vi "F Dwf Digital Can Rx.vi"(0 "hdwf":i32, 1 "pvID":i32, 2 "pfExtended":i32, 3 "pfRemote":i32, 4 "pcDLC":i32, 5 "rgRX":string, 6 "cRX":i32, 7 "error in (no error)":errorcluster, 8 "pvStatus":i32) -> (18 "pvStatus out":i32, 20 "function return":i32, 21 "pvID out":i32, 22 "pfExtended out":i32, 23 "pfRemote out":i32, 24 "pcDLC out":i32, 25 "rgRX out":string, 27 "error out":errorcluster)   [LabVIEW 2021, in "Olasdwf.lvlib"]
doc: "DWFAPI int FDwfDigitalCanRx(HDWF hdwf, int *pvID, int *pfExtended, int *pfRemote, int *pcDLC, unsigned char *rgRX, int cRX, int *pvStatus);"
uses:
  Olasdwf.lvlib
  Windows/System32/dwf.dll
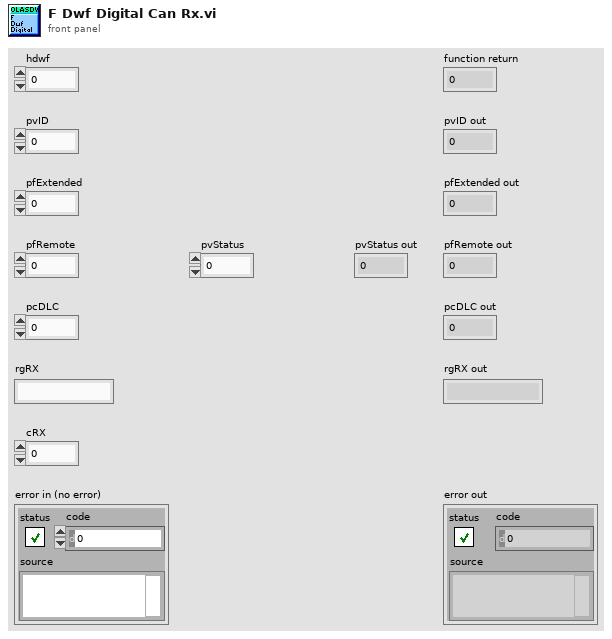
[diagram p1: front panel]
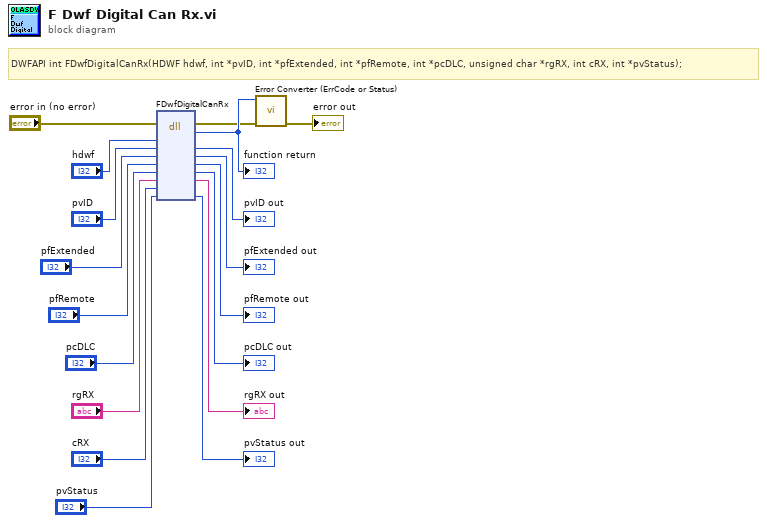
[diagram p0: block diagram]
diagram:
  # "DWFAPI int FDwfDigitalCanRx(HDWF hdwf, int *pvID, int *pfExtended, int *pfRemote, int *pcDLC, unsigned char *rgRX, int cRX, int *pvStatus);"
  n1 = dll-call lib="/Windows/System32/dwf.*" fn="FDwfDigitalCanRx"(error in="error in (no error)", "hdwf"="hdwf", "pvID"="pvID", "pfExtended"="pfExtended", "pfRemote"="pfRemote", "pcDLC"="pcDLC", "rgRX"="rgRX", "cRX"="cRX", "pvStatus"="pvStatus") -> (error out=w2:errorcluster, w18:i32, "pvID"=→"pvID out":i32, "pfExtended"=→"pfExtended out":i32, "pfRemote"=→"pfRemote out":i32, "pcDLC"=→"pcDLC out":i32, "rgRX"=→"rgRX out":string, "pvStatus"=→"pvStatus out":i32)  [unwired: 4 in, 1 out]
  "function return" <- w18
  n2 = call "Error Converter (ErrCode or Status).vi"("error in (no error)"=w2, "error code"=w18) -> ("error out"=→"error out":errorcluster)  [unwired: 9 in]
